vi "NT Build Topic Info from Names.vi"(11 "NT Topics":string[](array[string])) -> (3 "Topic Info":T1(array[cluster]))   [LabVIEW 2025]
uses:
  ntcoreffi.dll
  FRC_NetworkTablesLV.dll
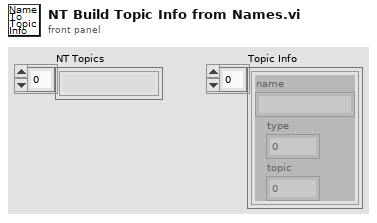
[diagram p1: front panel]
types:
  T1 = cluster{"name":string, "type":u32, "topic":u32}[]
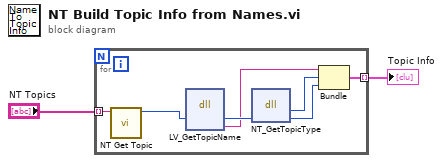
[diagram p0: block diagram]
diagram:
  n1 = for {
    tunnel: [w7] -> w1 mode=indexing
    tunnel: "NT Topics" -> [w5] mode=indexing
    n2 = call <vilib>:"NT Get Topic.vi"("name"=w5) -> ("topicHandle"=w4:u32)  [unwired: 9 in, 1 out]
    n3 = dll-call lib="FRC_NetworkTablesLV.*" fn="LV_GetTopicName"("topic"=w4) -> ("topic"=w9:u32, "name"=w3:string)  [unwired: 5 in, 2 out]
    n4 = dll-call lib="ntcoreffi.*" fn="NT_GetTopicType"("topic"=w9) -> ("type"=w8:u32, "topic"=w6:u32)  [unwired: 3 in, 2 out]
    n5 = Bundle("name"=w3, "type"=w8, "topic"=w6) -> (w7:cluster{"name":string, "type":u32, "topic":u32})  [unwired: 1 in]
  }
  "Topic Info" <- w1
